vi "Actor Core.vi"(8 "error in":errorcluster, 11 "4118 in":refnum<class "4118.lvclass">) -> (0 "error out":errorcluster, 3 "Actor out":refnum<class "Actor.lvclass">)   [LabVIEW 2024, in "4118 Actor.lvlib" / "4118.lvclass"]
doc: "<p>(<strong>Filename</strong>: <span class=\"dnl\">Actor Framework.lvlib:Actor.lvclass:Actor Core.vi</span>)</p>\n<p>Receives messages to the actor, reacts to them, and initiates any error handling that may shut the actor down.</p>\n<p>Descendant classes may override this VI to append parallel tasks for the actor to complete while it handles messages. Overrides use the <a href=\"nihelplauncher://docs/csh?context=lvcore_glang_udclass\">Call Parent Class Method</a> node.</p>"
uses:
  4118.lvclass
  C:/Program Files (x86)/National Instruments/LabVIEW 2024/vi.lib/ActorFramework/Actor/Actor.lvclass
  <vilib>/ActorFramework/Actor/Actor.lvclass
  4118.lvclass/4118.ctl
  <vilib>/ActorFramework/Actor/Actor.lvclass/Actor.ctl
  4118Func.ctl
  MFActor/ActorMessage/MF Task Name.ctl
  MFActor/NestedActorName.ctl
  MFActor/DeviceAlias.ctl
  MFActor/ActorMessage/MFActorMsg.lvclass
panel:
  in  "EndProc":bool
  out "MeasData":dbl[](array[numeric]) format="%.2f"
  out "UpdateData":bool
  out "In Query":bool
  out "Connected":bool
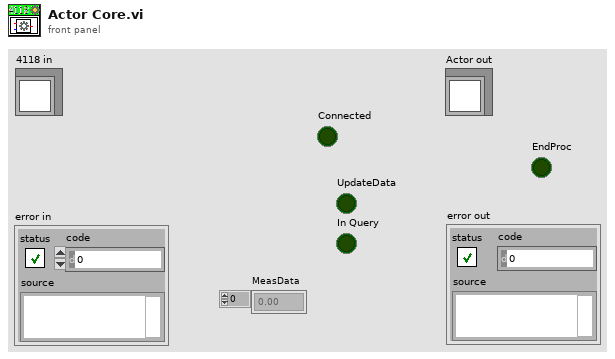
[diagram p1: front panel]
types:
  T1 = typedef "4118Func.ctl" = enum16{"④one", "Open", "Config", "Query", "ConvertData", "End"}
  T2 = cluster{"Interface":refnum<visa-resource-name>, "value range":string, "Channel Count":i32, "Limit 0":dbl, "Limit 1":dbl, "Limit 2":dbl, "Limit 3":dbl, "Limit 4":dbl, "Limit 5":dbl, "Limit 6":dbl, "Limit 7":dbl}
  T3 = cluster{"ManualFetchData":refnum<vi>, "AutoFetchData":refnum<vi>, "SampleRate":refnum<vi>}
  T4 = enum16{"Open", "Close", "Change Input Range", "Read Temp."}
  T5 = typedef "NestedActorName.ctl" = enum16{"None", "4503#0", "4503#1", "AIO#0", "AIO#1", "DIO", "PID", "TCPIP", "TestAngle", "TestFixPt", "TestMultiPt", "TestSinWave", "PW3390", "ADAM4118"}
  T6 = typedef "MF Task Name.ctl" = enum16{"DIChanged", "UpdateErrorCode", "SetTorque", "SetDriveTorque", "DataUpdated", "RunningTestProc", "StreamCtrl", "RunPID", "StopTest", "TCP Conn", "RefreshAutoUI", "ZeroAngle", "NestedActorLaunched", "NestedActorEnded", "ShowPsMsg"}
  T7 = enum16{"T/C Type J 0-760 ¢J", "T/C Type K 0-1370 ¢J", "T/C Type T -100-400 ¢J", "T/C Type E 0-1000 ¢J", "T/C Type R 500-1750 ¢J", "T/C Type S 500-1750 ¢J", "T/C Type B 500-1800 ¢J"}
  T8 = typedef "DeviceAlias.ctl" = enum16{"TQM0", "TQM1", "PM", "THERMO", "DC POWER"}
  T9 = cluster{"Temp.0[0]":dbl, "Temp.0[1]":dbl, "Temp.0[2]":dbl, "Temp.0[3]":dbl, "Temp.0[4]":dbl, "Temp.0[5]":dbl, "Temp.0[6]":dbl, "Temp.0[7]":dbl}
  T10 = cluster{"MF Msg Enum":T6, cluster{"MeasData":dbl[], "Device":T8}}
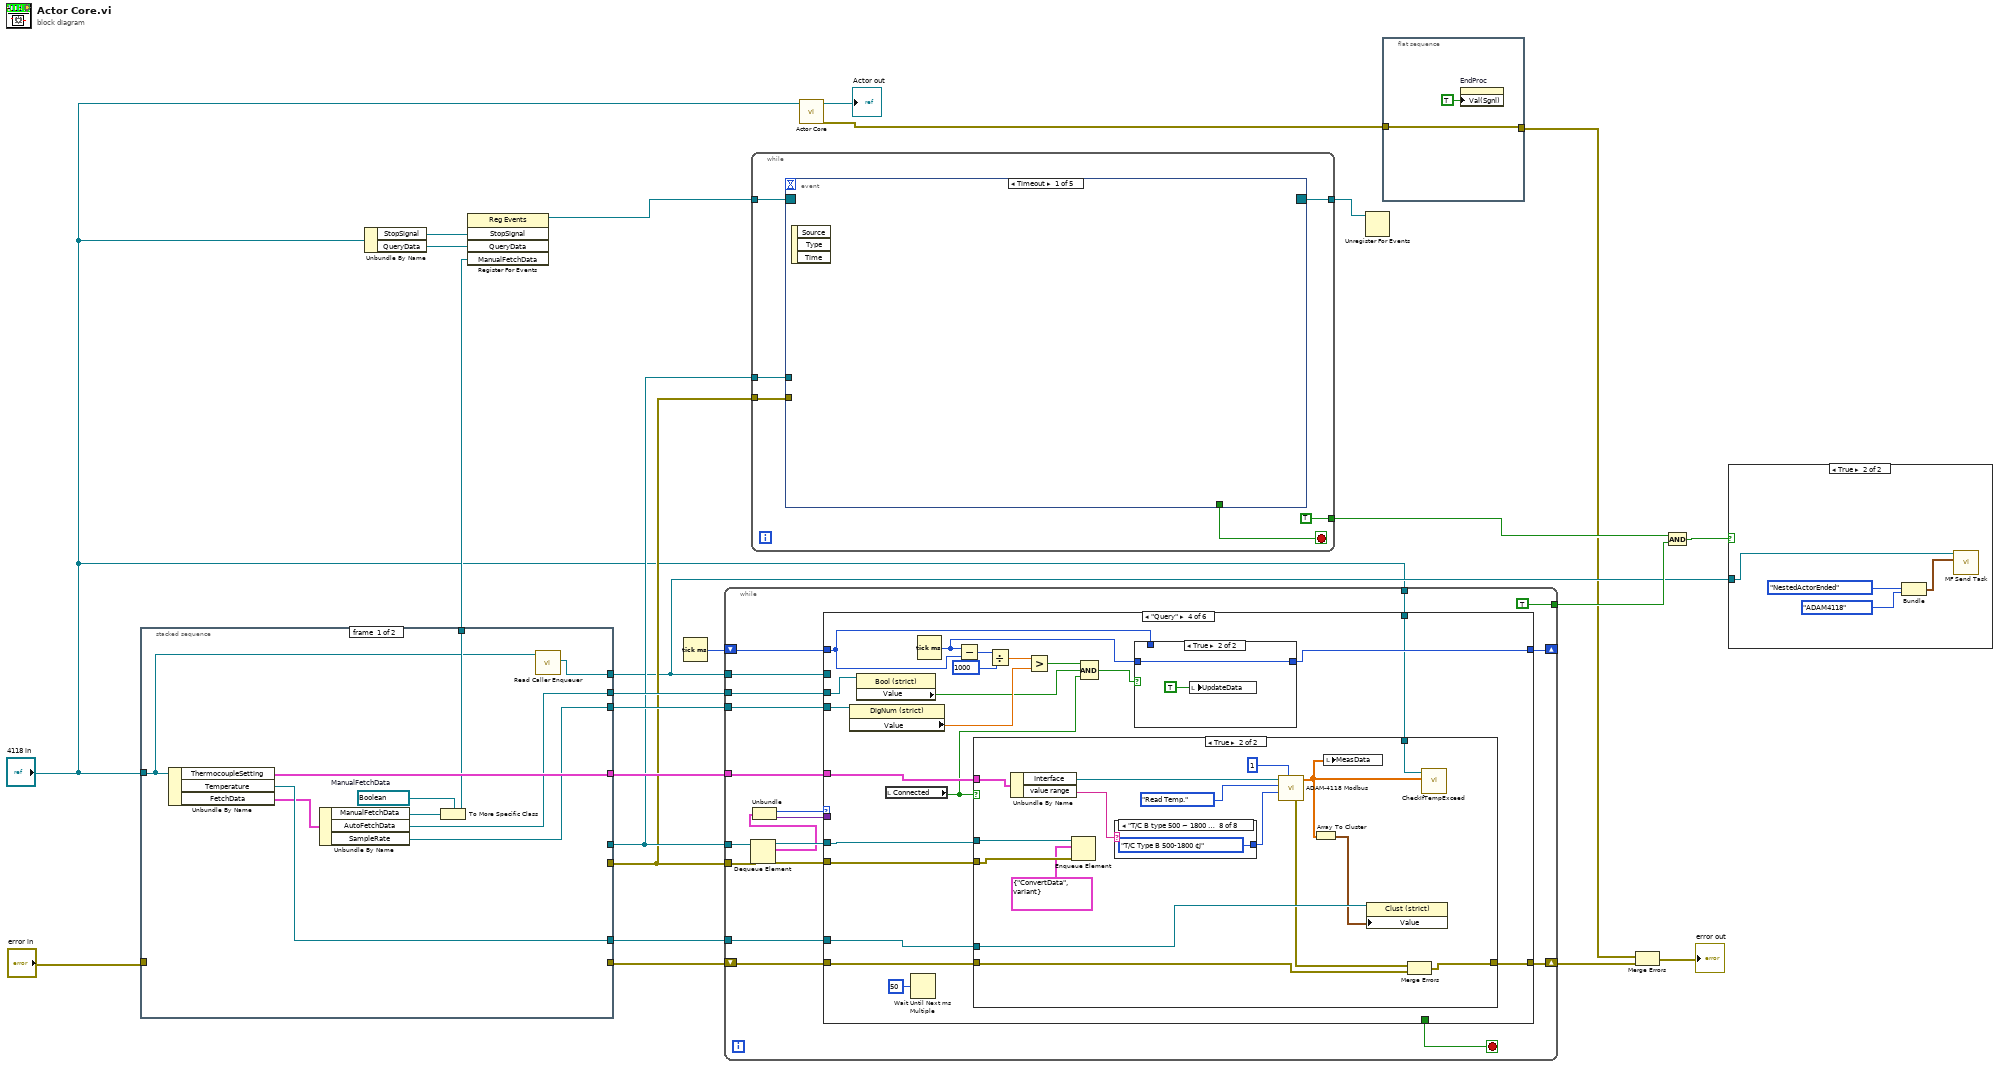
[diagram p0: block diagram]
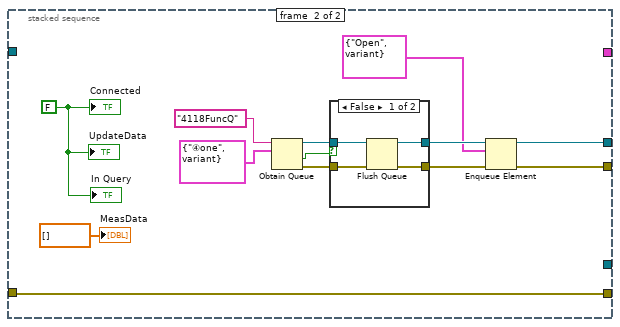
[diagram p3: hidden frame]
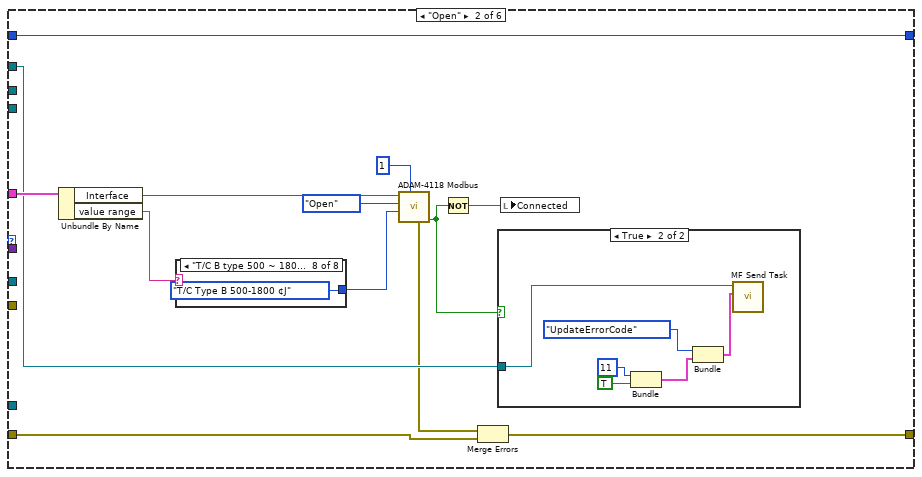
[diagram p6: hidden frame]
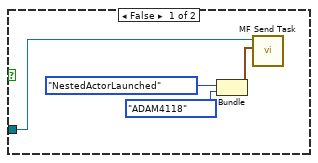
[diagram p7: hidden frame]
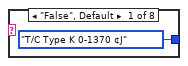
[diagram p8: hidden frame]
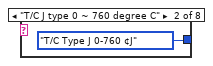
[diagram p9: hidden frame]
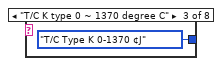
[diagram p10: hidden frame]
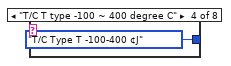
[diagram p11: hidden frame]
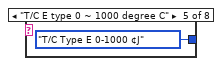
[diagram p12: hidden frame]
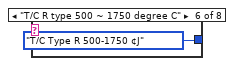
[diagram p13: hidden frame]
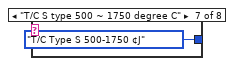
[diagram p14: hidden frame]
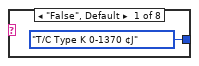
[diagram p18: hidden frame]
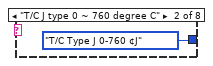
[diagram p19: hidden frame]
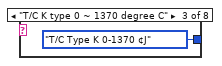
[diagram p20: hidden frame]
diagram:
  n1 = stacked-sequence {
    tunnel: "4118 in" -> [w26 _]
    tunnel: "error in" -> [_ w35]
    tunnel: [w34 _] -> w18
    tunnel: [w33 _] -> w17
    tunnel: [w30 _] -> w16
    tunnel: [w29 _] -> w15
    tunnel: [w28 _] -> w14
    tunnel: [_ w39] -> w13
    tunnel: [_ w38] -> w12
    tunnel: [w25 _] -> w4
    tunnel: [_ w35] -> w10
    frame #0 {
      w27 = refnum<vi> refnum  # ManualFetchData
      n2 = Unbundle By Name(w26) -> ("ThermocoupleSetting"=w34:T2, "Temperature"=w33:refnum<vi>, "FetchData"=w32:T3)
      n3 = Unbundle By Name(w32) -> ("ManualFetchData"=w31:refnum<vi>, "AutoFetchData"=w29:refnum<vi>, "SampleRate"=w28:refnum<vi>)
      n4 = To More Specific Class(target class=w27, reference=w31) -> (specific class reference=w30:refnum<vi>)  [unwired: 1 in, 1 out]
      n5 = call <vilib>:"Read Caller Enqueuer.vi"("Actor"=w26) -> ("Caller Enqueuer"=w25:refnum<class "Message Enqueuer.lvclass">)  [unwired: 10 in]
    }
    frame #1 {
      w37 = FALSE ("Connected")
      n6 = Obtain Queue(name (unnamed)="4118FuncQ", element data type=cluster{"4118Func":T1, variant} {"4118Func"=enum."④one", variant}) -> (queue out=w45:refnum<queue>, created new?=w43:bool, error out=w44:errorcluster)  [unwired: 3 in]
      n7 = case shown="False" w43 {
        tunnel: w45 -> [w51 w53]
        tunnel: w44 -> [w50 w52]
        tunnel: [w49 w53] -> w42
        tunnel: [w48 w52] -> w41
        frame False {
          n8 = Flush Queue(queue=w51, error in (no error)=w50) -> (queue out=w49:refnum<queue>, error out=w48:errorcluster)  [unwired: 1 out]
        }
        frame True {
        }
      }
      n9 = Enqueue Element(queue=w42, element=cluster{"4118Func":T1, variant} {"4118Func"=enum."Open", variant}, error in (no error)=w41) -> (queue out=w39:refnum<queue>, error out=w38:errorcluster)  [unwired: 1 in, 1 out]
      "Connected" <- w37
      "UpdateData" <- w37
      "In Query" <- w37
      "MeasData" <- dbl[] [] ("MeasData")
    }
  }
  n10 = Unbundle By Name("4118 in") -> ("StopSignal"=w21:refnum<user-event>, "QueryData"=w20:refnum<user-event>)
  n11 = register-events(w21, w20, w16) -> (reference out=w19:refnum<event-registration>)  [unwired: 2 in, 1 out]
  n12 = Tick Count (ms)() -> (millisecond timer value=w11:u32)
  n13 = while {
    tunnel: w18 -> [w62]
    tunnel: w17 -> [w60]
    tunnel: w15 -> [w64]
    tunnel: w14 -> [w63]
    tunnel: w13 -> [w71]
    tunnel: w12 -> [w72]
    tunnel: w4 -> [w61]
    shift-right: [w58] -> _
    shift-left: w11 -> [w59]
    shift-right: [w57] -> w9
    shift-left: w10 -> [w56]
    tunnel: [TRUE] -> w6
    tunnel: "4118 in" -> [w54]
    stop <- w65 stop-if-true
    n14 = Dequeue Element(queue=w71, error in (no error)=w72) -> (queue out=w70:refnum<queue>, element=w68:cluster{"4118Func":T1, variant}, error out=w69:errorcluster)  [unwired: 1 in, 1 out]
    n15 = Unbundle(w68) -> ("4118Func"=w67:T1, w66:variant)
    n16 = case shown="\"Query\"" w67 {
      tunnel: w70 -> [_ _ _ w113 w161 w181]
      tunnel: w69 -> [_ _ _ w112 w160 w180]
      tunnel: w66 -> [_ _ _ _ _ _]
      tunnel: [_ _ _ _ _ TRUE] -> w65
      tunnel: w64 -> [_ _ _ w120 _ _]
      tunnel: w63 -> [_ _ _ w123 _ _]
      tunnel: w62 -> [_ w86 _ w128 _ _]
      tunnel: w61 -> [_ w81 _ _ w158 _]
      tunnel: w60 -> [_ _ _ w127 _ _]
      tunnel: w59 -> [w74 w78 w107 w116 w163 w176]
      tunnel: [w74 w78 w107 w114 w163 w176] -> w58
      tunnel: [w73 w76 w106 w110 w157 w174] -> w57
      tunnel: w56 -> [w73 w77 w106 w111 w157 w174]
      tunnel: w54 -> [_ _ _ w108 _ _]
      frame "④one", Default {
      }
      frame "Open" {
        n17 = Unbundle By Name(w86) -> ("Interface"=w85:refnum<visa-resource-name>, "value range"=w83:string)
        n18 = case shown="\"T/C B type 500 ~ 1800 degree C\"" w83 {
          tunnel: [T7."T/C Type K 0-1370 ¢J" ("Input Range") T7."T/C Type J 0-760 ¢J" ("Input Range") T7."T/C Type K 0-1370 ¢J" ("Input Range") T7."T/C Type T -100-400 ¢J" ("Input Range") T7."T/C Type E 0-1000 ¢J" ("Input Range") T7."T/C Type R 500-1750 ¢J" ("Input Range") T7."T/C Type S 500-1750 ¢J" ("Input Range") T7."T/C Type B 500-1800 ¢J" ("Input Range")] -> w82
          frame "False", Default {
          }
          frame "T/C J type 0 ~ 760 degree C" {
          }
          frame "T/C K type 0 ~ 1370 degree C" {
          }
          frame "T/C T type -100 ~ 400 degree C" {
          }
          frame "T/C E type 0 ~ 1000 degree C" {
          }
          frame "T/C R type 500 ~ 1750 degree C" {
          }
          frame "T/C S type 500 ~ 1750 degree C" {
          }
          frame "T/C B type 500 ~ 1800 degree C" {
          }
        }
        n19 = call "ADAM-4118 Modbus.vi"("CardCount"=1, "Input Range"=w82, "Function"=T4."Open", "VISA resource name"=w85) -> ("Error"=w80:bool, "error out"=w75:errorcluster)  [unwired: 3 in, 3 out]
        n20 = Not(x=w80) -> (.not. x?=w79:bool)
        n21 = Merge Errors(w75, w77) -> (w76:errorcluster)
        n22 = case shown="True" w80 {
          tunnel: w81 -> [w91 w97]
          frame False {
            n23 = Bundle("MF Msg Enum"=MF_Task_Name."NestedActorLaunched", "NestedActorName"=NestedActorName."ADAM4118") -> (w88:cluster{"MF Msg Enum":T6, "NestedActorName":T5})  [unwired: 1 in]
            n24 = call "MF Send Task.vi"("MsgType"=w88, "Message Enqueuer"=w91) -> ()  [unwired: 9 in, 1 out]
          }
          frame True {
            n25 = Bundle(11, TRUE) -> (w95:cluster{i32, bool})  [unwired: 1 in]
            n26 = Bundle("MF Msg Enum"=MF_Task_Name."UpdateErrorCode", w95) -> (w92:cluster{"MF Msg Enum":T6, cluster{i32, bool}})  [unwired: 1 in]
            n27 = call "MF Send Task.vi"("MsgType"=w92, "Message Enqueuer"=w97) -> ()  [unwired: 9 in, 1 out]
          }
        }
        n28 = local write "Connected"(w79) -> ()
      }
      frame "Config" {
      }
      frame "Query" {
        n29 = property class="DigNum (strict)"(reference=w123) -> ("Value"=w122:dbl)  [unwired: 1 in, 2 out]
        n30 = property class="Bool (strict)"(reference=w120) -> ("Value"=w119:bool)  [unwired: 1 in, 2 out]
        n31 = local read "Connected"() -> (w118:bool)
        n32 = Wait Until Next ms Multiple(millisecond multiple=u32 50) -> ()  [unwired: 1 out]
        n33 = Tick Count (ms)() -> (millisecond timer value=w115:u32)
        n34 = Subtract(x=w115, y=w116) -> (x-y=w126:u32)
        n35 = case shown="True" w118 {
          tunnel: w128 -> [_ w148]
          tunnel: w127 -> [_ w142]
          tunnel: w113 -> [_ w140]
          tunnel: w112 -> [_ w139]
          tunnel: w111 -> [w132 w136]
          tunnel: [w132 w135] -> w110
          tunnel: w108 -> [_ w134]
          frame False {
          }
          frame True {
            n36 = Unbundle By Name(w148) -> ("Interface"=w147:refnum<visa-resource-name>, "value range"=w145:string)
            n37 = Enqueue Element(queue=w140, element=cluster{"4118Func":T1, variant} {"4118Func"=enum."ConvertData", variant}, error in (no error)=w139) -> ()  [unwired: 1 in, 3 out]
            n38 = case shown="\"T/C B type 500 ~ 1800 degree C\"" w145 {
              tunnel: [T7."T/C Type K 0-1370 ¢J" ("Input Range") T7."T/C Type J 0-760 ¢J" ("Input Range") T7."T/C Type K 0-1370 ¢J" ("Input Range") T7."T/C Type T -100-400 ¢J" ("Input Range") T7."T/C Type E 0-1000 ¢J" ("Input Range") T7."T/C Type R 500-1750 ¢J" ("Input Range") T7."T/C Type S 500-1750 ¢J" ("Input Range") T7."T/C Type B 500-1800 ¢J" ("Input Range")] -> w144
              frame "False", Default {
              }
              frame "T/C J type 0 ~ 760 degree C" {
              }
              frame "T/C K type 0 ~ 1370 degree C" {
              }
              frame "T/C T type -100 ~ 400 degree C" {
              }
              frame "T/C E type 0 ~ 1000 degree C" {
              }
              frame "T/C R type 500 ~ 1750 degree C" {
              }
              frame "T/C S type 500 ~ 1750 degree C" {
              }
              frame "T/C B type 500 ~ 1800 degree C" {
              }
            }
            n39 = call "ADAM-4118 Modbus.vi"("CardCount"=1, "Input Range"=w144, "Function"=T4."Read Temp.", "VISA resource name"=w147) -> ("Temp.0"=w133:dbl[], "error out"=w137:errorcluster)  [unwired: 3 in, 3 out]
            n40 = Array To Cluster(array=w133) -> (cluster=w141:T9)
            n41 = local write "MeasData"(w133) -> ()
            n42 = property class="Clust (strict)"(reference=w142, "Value"=w141) -> ()  [unwired: 1 in, 2 out]
            n43 = Merge Errors(w137, w136) -> (w135:errorcluster)
            n44 = call "CheckIfTempExceed.vi"("MeasData"=w133, "4118 in"=w134) -> ()  [unwired: 8 in, 2 out]
          }
        }
        n45 = Divide(x=w126, y=u32 1000) -> (x/y=w124:dbl)
        n46 = Greater?(x=w124, y=w122) -> (0:w121:bool)
        n47 = Compound Arithmetic op=AND(w121, w119, w118) -> (w117:bool)
        n48 = case shown="True" w117 {
          tunnel: w116 -> [w129 _]
          tunnel: w115 -> [_ w130]
          tunnel: [w129 w130] -> w114
          frame False {
          }
          frame True {
            n49 = local write "UpdateData"(TRUE) -> ()
          }
        }
      }
      frame "ConvertData" {
        n50 = local read "In Query"() -> (w162:bool)
        n51 = local read "UpdateData"() -> (w159:bool)
        n52 = case shown="True" w159 {
          tunnel: w158 -> [_ w170]
          frame False {
          }
          frame True {
            n53 = local read "MeasData"() -> (w166:dbl[])
            n54 = Bundle("MeasData"=w166, "Device"=DeviceAlias."THERMO") -> (w167:cluster{"MeasData":dbl[], "Device":T8})  [unwired: 1 in]
            n55 = Bundle("MF Msg Enum"=MF_Task_Name."DataUpdated", w167) -> (w165:T10)  [unwired: 1 in]
            n56 = local write "UpdateData"(FALSE) -> ()
            n57 = call "MF Send Task.vi"("MsgType"=w165, "Message Enqueuer"=w170) -> ()  [unwired: 9 in, 1 out]
          }
        }
        n58 = case shown="True" w162 {
          tunnel: w161 -> [_ w173]
          tunnel: w160 -> [_ w172]
          frame False {
          }
          frame True {
            n59 = Enqueue Element(queue=w173, element=cluster{"4118Func":T1, variant} {"4118Func"=enum."Query", variant}, error in (no error)=w172) -> ()  [unwired: 1 in, 3 out]
          }
        }
      }
      frame "End" {
        n60 = Flush Queue(queue=w181, error in (no error)=w180) -> (queue out=w179:refnum<queue>, error out=w178:errorcluster)  [unwired: 1 out]
        n61 = Release Queue(queue=w179, error in (no error)=w178) -> ()  [unwired: 1 in, 3 out]
        n62 = call "ADAM-4118 Modbus.vi"("Function"=T4."Close") -> ()  [unwired: 6 in, 5 out]
      }
    }
  }
  n63 = while {
    tunnel: [w187] -> w23
    tunnel: w19 -> [w186]
    tunnel: w13 -> [w184]
    tunnel: w12 -> [w183]
    tunnel: [TRUE] -> w7
    stop <- w185 stop-if-true
    n64 = event shown="[0] Timeout" {
      selector: w186 -> [_ _ _ _ _]
      dyn-events: [_ _ _ _ _] -> w187
      timeout: _ -> [_ _ _ _ _]
      tunnel: [_ "EndProc" _ _ _] -> w185
      tunnel: w184 -> [_ _ w194 w196 _]
      tunnel: w183 -> [_ _ w193 w195 _]
      event Timeout {
        n65 = event-data() -> ()  [unwired: 1 in, 3 out]
      }
      event "EndProc": Value Change {
        n66 = event-data() -> ()  [unwired: 1 in, 6 out]
      }
      event User Event {
        w189 = FALSE ("Connected")
        n67 = event-data() -> ()  [unwired: 1 in, 5 out]
        n68 = Flush Queue(queue=w194, error in (no error)=w193) -> (queue out=w192:refnum<queue>, error out=w191:errorcluster)  [unwired: 1 out]
        n69 = Enqueue Element At Opposite End(queue=w192, element=cluster{"4118Func":T1, variant} {"4118Func"=enum."End", variant}, error in (no error)=w191) -> ()  [unwired: 1 in, 3 out]
        n70 = local write "Connected"(w189) -> ()
        n71 = local write "UpdateData"(w189) -> ()
        n72 = local write "In Query"(w189) -> ()
      }
      event User Event {
        n73 = event-data() -> ("QueryData"=w197:bool)  [unwired: 1 in, 4 out]
        n74 = case shown="True" w197 {
          selector: w197 -> [w198 _]
          tunnel: w196 -> [_ w200]
          tunnel: w195 -> [_ w199]
          frame False {
            n75 = local write "In Query"(w198) -> ()
          }
          frame True {
            n76 = local read "In Query"() -> (w201:bool)
            n77 = case shown="False" w201 {
              tunnel: w200 -> [w204 _]
              tunnel: w199 -> [w203 _]
              frame False {
                n78 = local write "In Query"(TRUE) -> ()
                n79 = Enqueue Element(queue=w204, element=cluster{"4118Func":T1, variant} {"4118Func"=enum."Query", variant}, error in (no error)=w203) -> ()  [unwired: 1 in, 3 out]
              }
              frame True {
              }
            }
          }
        }
      }
      event Value Change {
        n80 = event-data() -> ()  [unwired: 1 in, 6 out]
        n81 = local write "UpdateData"(TRUE) -> ()
      }
    }
  }
  n82 = call-parent "Actor Core.vi"("Actor in"="4118 in") -> ("error out"=w2:errorcluster, "Actor out"=→"Actor out":refnum<class "Actor.lvclass">)  [unwired: 9 in]
  n83 = Unregister For Events(event registration refnum=w23) -> ()  [unwired: 1 in, 1 out]
  n84 = flat-sequence {
    tunnel: w2 -> [w208]
    tunnel: [w208] -> w1
    frame #0 {
      n85 = property on="EndProc" class="Bool (strict)"("Val(Sgnl)"=TRUE ("Value (Signaling)")) -> ()  [unwired: 2 in, 2 out]
    }
  }
  n86 = Merge Errors(w1, w9) -> (→"error out":errorcluster)
  n87 = Compound Arithmetic op=AND(w7, w6) -> (w5:bool)
  n88 = case shown="True" w5 {
    tunnel: w4 -> [_ w209]
    frame False {
    }
    frame True {
      n89 = Bundle("MF Msg Enum"=MF_Task_Name."NestedActorEnded", "NestedActorName"=NestedActorName."ADAM4118") -> (w210:cluster{"MF Msg Enum":T6, "NestedActorName":T5})  [unwired: 1 in]
      n90 = call "MF Send Task.vi"("MsgType"=w210, "Message Enqueuer"=w209) -> ()  [unwired: 9 in, 1 out]
    }
  }
